vi "NanonisProperties_rawspeed.vi"(0 "Application ref in":refnum<vi>, 5 "Position":cluster{"X":dbl, "Y":dbl, "Z pen":dbl, "Z":dbl}, 11 "error in (no error)":errorcluster, 12 "Z Write?":bool, 13 "XY Write?":bool=TRUE) -> (4 "Application ref out":refnum<vi>, 15 "error out":errorcluster)   [LabVIEW 2019]
uses:
  <userlib>/Nanonis Prog Interface V5/Nanonis Prog Interface.lvlib
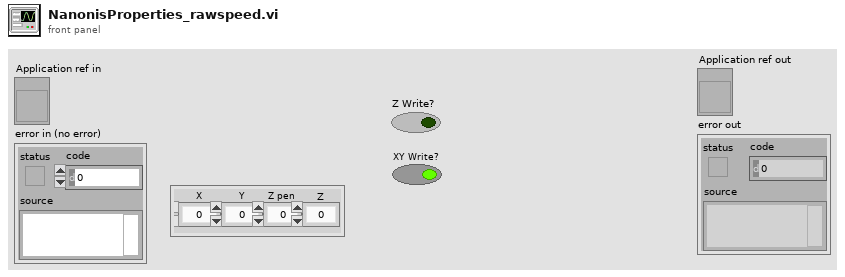
[diagram p1: front panel]
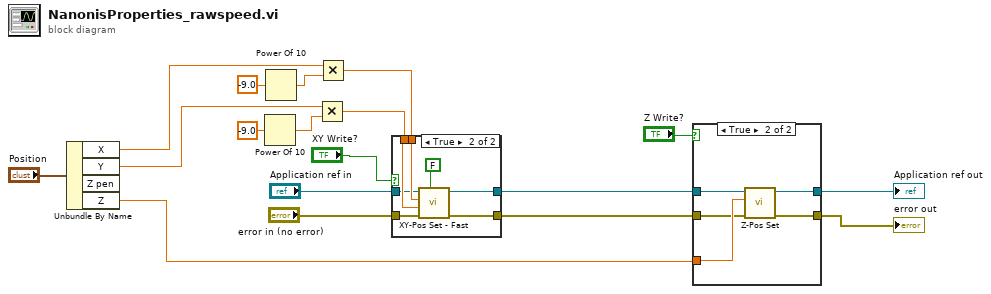
[diagram p0: block diagram]
diagram:
  n1 = Unbundle By Name("Position") -> ("X"=w3:dbl, "Y"=w2:dbl, "Z"=w1:dbl)  [unwired: 1 out]
  n2 = Power Of 10(x=-9.0) -> (10^x=w16:dbl)
  n3 = Power Of 10(x=-9.0) -> (10^x=w18:dbl)
  n4 = Multiply(x=w2, y=w16) -> (x*y=w13:dbl)
  n5 = Multiply(x=w3, y=w18) -> (x*y=w14:dbl)
  n6 = case shown="True" "XY Write?" {
    tunnel: w14 -> [_ w26]
    tunnel: w13 -> [_ w25]
    tunnel: "Application ref in" -> [w20 w24]
    tunnel: "error in (no error)" -> [w19 w23]
    tunnel: [w20 w22] -> w7
    tunnel: [w19 w21] -> w6
    frame False {
    }
    frame True {
      n7 = call <userlib>:"XY-Pos Set - Fast.vi"("Wait end-of-motion (T=True)"=FALSE, "error in (no error)"=w23, "Y (m)"=w25, "X (m)"=w26, "Application ref in"=w24) -> ("error out"=w21:errorcluster, "Application ref out"=w22:refnum<vi>)  [unwired: 4 in]
    }
  }
  n8 = case shown="True" "Z Write?" {
    tunnel: w7 -> [w29 w34]
    tunnel: [w29 w33] -> w12
    tunnel: [w28 w32] -> w11
    tunnel: w1 -> [_ w31]
    tunnel: w6 -> [w28 w30]
    frame False {
    }
    frame True {
      n9 = call <userlib>:"Z-Pos Set.vi"("error in (no error)"=w30, "Z position (m)"=w31, "Application ref in"=w34) -> ("error out"=w32:errorcluster, "Application ref out"=w33:refnum<vi>)  [unwired: 7 in]
    }
  }
  "Application ref out" <- w12
  "error out" <- w11
